vi "Write DCLinkSteadyState.vi"(8 "error in (no error)":errorcluster, 10 "DCLinkSteadyState":dbl, 11 "AppStateMachine configuration in":refnum<class "AppStateMachine configuration.lvclass">) -> (0 "error out":errorcluster, 3 "AppStateMachine configuration out":refnum<class "AppStateMachine configuration.lvclass">)   [LabVIEW 2017, in "AppStateMachine configuration.lvclass"]
uses:
  AppStateMachine configuration.lvclass
  AppStateMachine configuration.lvclass/AppStateMachine configuration.ctl
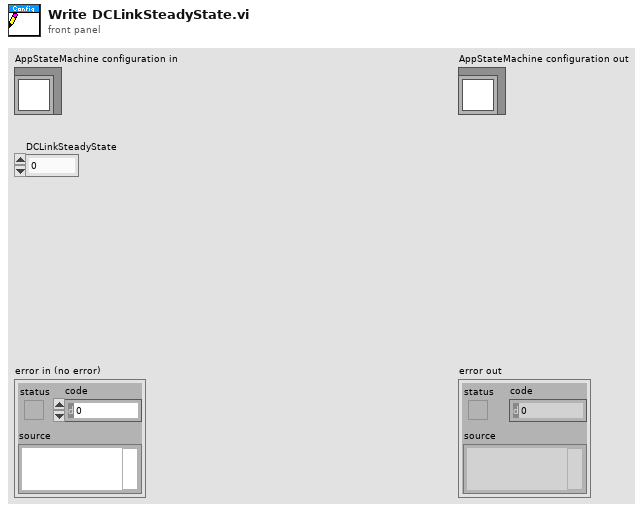
[diagram p1: front panel]
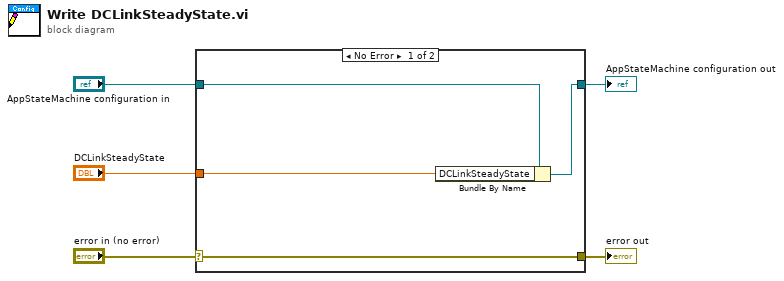
[diagram p0: block diagram]
diagram:
  n1 = case shown="No Error" "error in (no error)" {
    selector: "error in (no error)" -> [w9 w10]
    tunnel: [w9 w10] -> w4
    tunnel: [w7 w11] -> w2
    tunnel: "AppStateMachine configuration in" -> [w8 w11]
    tunnel: "DCLinkSteadyState" -> [w6 _]
    frame No Error {
      n2 = Bundle By Name(cluster=w8, "DCLinkSteadyState"=w6) -> (w7:refnum<class "AppStateMachine configuration.lvclass">)
    }
    frame Error {
    }
  }
  "error out" <- w4
  "AppStateMachine configuration out" <- w2
